vi "WaitForCamera.vi"(2 "error in":errorcluster, 3 "QT Ref In":T1) -> (0 "error out":errorcluster, 1 "QT Ref Out":T1)   [LabVIEW 2010]
uses:
  <userlib>/ImageProcessing/QTLIB_2595_LV86/QT_Ref.ctl
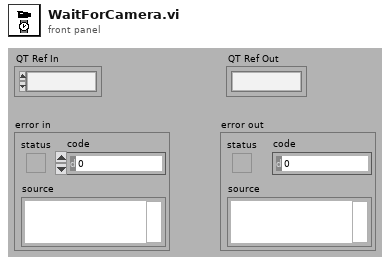
[diagram p1: front panel]
types:
  T1 = typedef "QT_Ref.ctl" = refnum<k1>
  T2 = typedef "QT_Image.ctl" = cluster{"Width":i32, "Height":i32, "Depth":i32, "data":u8[], "Compressed data":u8[], "Color table":u32[], "Duration":i32, "Options":i32, "Timestamp":i32, "ID":i32, "Reserved":i32, "Dialogs":u32}
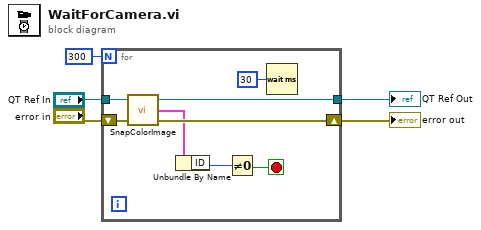
[diagram p0: block diagram]
diagram:
  n1 = for {
    N: 300 -> [_]
    tunnel: "QT Ref In" -> [w13]
    shift-right: [w11] -> w4
    shift-left: "error in" -> [w12]
    tunnel: [w10] -> w5
    stop <- w7 stop-if-true
    n2 = call <userlib>:"SnapColorImage.vi"("error in (no error)"=w12, "QT Ref In"=w13) -> ("error out"=w11:errorcluster, "Image Out"=w8:T2, "QT Ref Out"=w10:T1)  [unwired: 1 in]
    n3 = Unbundle By Name(w8) -> ("ID"=w6:i32)
    n4 = Not Equal To 0?(x=w6) -> (x != 0?=w7:bool)
    n5 = Wait (ms)(milliseconds to wait=u32 30) -> ()  [unwired: 1 out]
  }
  "QT Ref Out" <- w5
  "error out" <- w4
